vi "SaneVelocities.vi"(8 "Probe Type":u16(ring)=12 items=["5-Hole Probe"=5, "OmniProbe"=12], 10 "DataIn":T1) -> (0 "VelocityErrors":T2={"PressureErrors"=[], "Plug in titles"=["Good", "AllNegative", "dPTooSmall", "P1smallest", "FailedToReduce", "ExceedMaxCone", "U.LT.0"]}, 2 "DataOut":T1)   [LabVIEW 2016]
doc: "Removes samples- shortening output array- which do not satisfy sanity checks:\nCone angle should be within probe's range;\n5HP velocity should be >0, Omniprobe, arbitrarily, -30m/s;\nIndividual measurements should be within prescribed sigma of that component's mean."
uses:
  SanityCluster.ctl
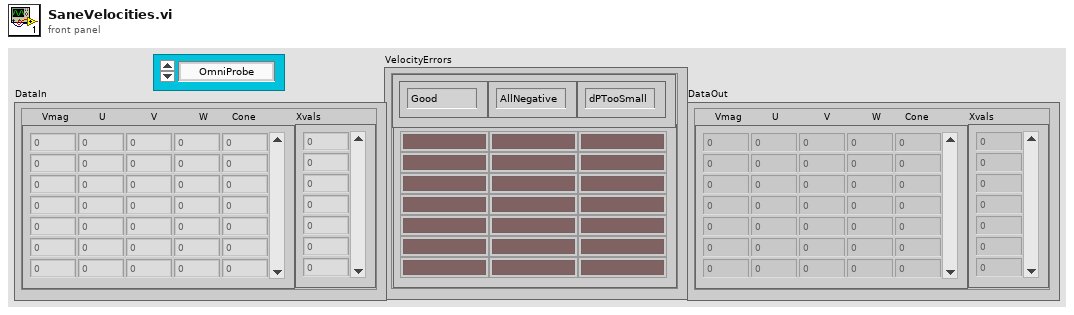
[diagram p1: front panel]
types:
  T1 = cluster{"   Vmag          U               V              W        Cone":dbl[][], "Xvals":i32[]}
  T2 = typedef "SanityCluster.ctl" = cluster{"PressureErrors":bool[][], "Plug in titles":string[]}
  T3 = cluster{"   Vmag          U               V              W        Cone":dbl[][], i32[]}
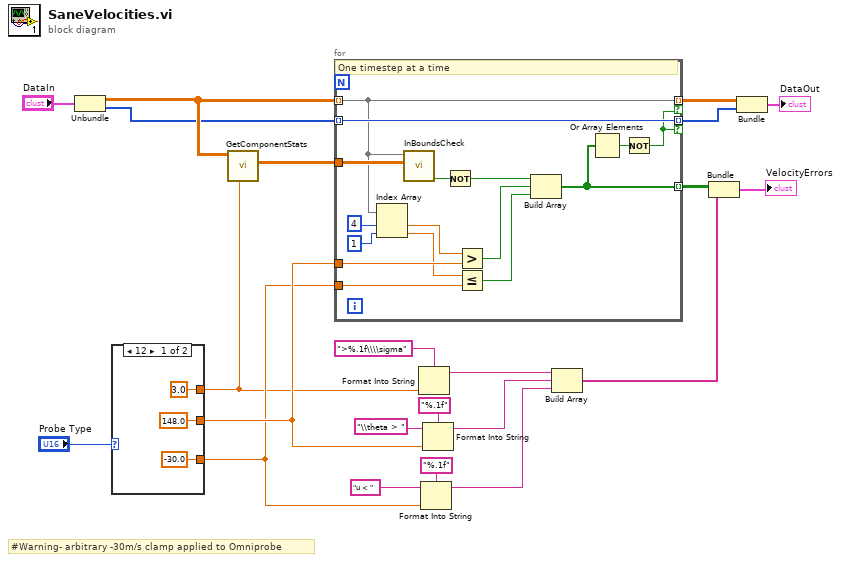
[diagram p0: block diagram]
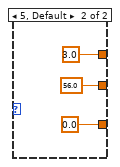
[diagram p2: hidden frame]
diagram:
  # "#Warning- arbitrary -30m/s clamp applied to Omniprobe"
  n1 = Unbundle("DataIn") -> ("Vmag          U               V              W        Cone"=w5:dbl[][], "Xvals"=w4:i32[])
  n2 = case shown="12" "Probe Type" {
    tunnel: [148.0 ("MaxCone") 56.0 ("MaxCone")] -> w12
    tunnel: [-30.0 ("Umin") 0.0 ("Umin")] -> w11
    tunnel: [3.0 ("+/-sigmaBounds") 3.0 ("+/-sigmaBounds")] -> w7
    frame 12 {
    }
    frame 5, Default {
    }
  }
  n3 = call "GetComponentStats.vi"("+/-sigmaBounds"=w7, "Vmag         U             V             W          Cone"=w5) -> ("Stats"=w10:dbl[][])  [unwired: 9 in]
  n4 = for {
    tunnel: [w44] -> w16 mode=indexing
    tunnel: w11 -> [w41]
    tunnel: w12 -> [w40]
    tunnel: [w33] -> w3 mode=indexing if=w37
    tunnel: w5 -> [w33] mode=indexing
    tunnel: [w38] -> w2 mode=indexing if=w37
    tunnel: w4 -> [w38] mode=indexing
    tunnel: w10 -> [w36]
    # "One timestep at a time"
    n5 = Index Array(array=w33, index #1=4 ("disabled index (col)"), index #2=1 ("index (col)")) -> (element #1=w30:dbl, element #2=w29:dbl)
    n6 = call "InBoundsCheck.vi"("Stats in"=w36, "RawVmagUVWCone in"=w33) -> ("allGood"=w35:bool)  [unwired: 9 in]
    n7 = Not(x=w35) -> (.not. x?=w34:bool)
    n8 = Greater?(x=w30, y=w40) -> (0:w43:bool)
    n9 = Less Or Equal?(x=w29, y=w41) -> (x <= y?=w42:bool)
    n10 = Build Array(w34, w43, w42) -> (w44:bool[])
    n11 = Or Array Elements(Boolean array=w44) -> (logical OR=w39:bool)
    n12 = Not(x=w39) -> (.not. x?=w37:bool)
  }
  n13 = Format Into String(format string=">%.1f\\\\sigma", w7) -> (resulting string=w8:string)  [unwired: 2 in, 1 out]
  n14 = Format Into String(format string="%.1f", initial string="u < ", w11) -> (resulting string=w17:string)  [unwired: 1 in, 1 out]
  n15 = Format Into String(format string="%.1f", initial string="\\theta > ", w12) -> (resulting string=w20:string)  [unwired: 1 in, 1 out]
  n16 = Build Array(w8, w20, w17) -> (w15:string[])
  n17 = Bundle(w16, w15) -> (→"VelocityErrors":cluster{bool[][], string[]})  [unwired: 1 in]
  n18 = Bundle("Vmag          U               V              W        Cone"=w3, w2) -> (→"DataOut":T3)  [unwired: 1 in]
